vi "Create Library Folder.vi"(11 "Second Library Script Strategy in":refnum<class "Second Library Script Strategy.lvclass">) -> (2 "Library Folder Already Exists?":bool, 3 "Second Library Script Strategy out":refnum<class "Second Library Script Strategy.lvclass">)   [LabVIEW 2021, in "_Create From Template.lvlib" / "Script Strategy.lvlib" / "Second Library Script Strategy.lvclass"]
uses:
  Second Library Script Strategy.lvclass
  Second Library Script Strategy.lvclass/Second Library Script Strategy.ctl
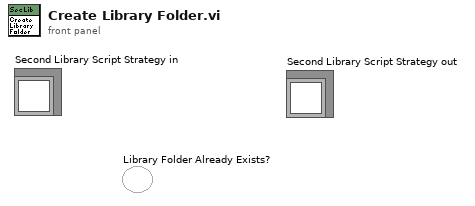
[diagram p1: front panel]
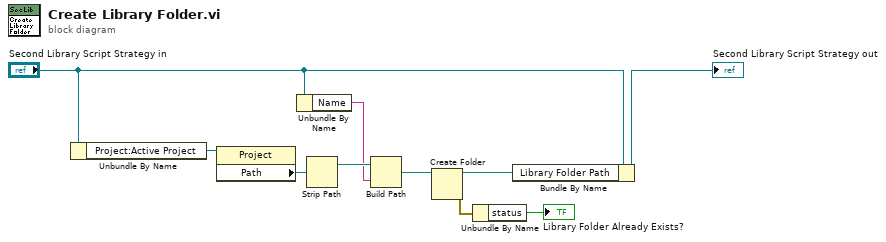
[diagram p0: block diagram]
diagram:
  n1 = Unbundle By Name("Second Library Script Strategy in") -> ("Project:Active Project"=w3:refnum<vi>)
  n2 = property class="Project"(reference=w3) -> ("Path"=w8:path)  [unwired: 1 in, 2 out]
  n3 = Unbundle By Name("Second Library Script Strategy in") -> ("Name"=w5:string)
  n4 = Strip Path(path=w8) -> (stripped path=w9:path)  [unwired: 1 out]
  n5 = Build Path(base path=w9, name or relative path=w5) -> (appended path=w10:path)
  n6 = Create Folder(path (use dialog)=w10) -> (created path=w1:path, error out=w7:errorcluster)  [unwired: 2 in, 1 out]
  n7 = Unbundle By Name(w7) -> ("status"=→"Library Folder Already Exists?":bool)
  n8 = Bundle By Name(cluster="Second Library Script Strategy in", "Library Folder Path"=w1) -> (→"Second Library Script Strategy out":refnum<class "Second Library Script Strategy.lvclass">)
